vi "Actor Core.vi"(8 "error in":errorcluster, 11 "SLZ-KA1 in":refnum<class "SLZ-KA1.lvclass">) -> (0 "error out":errorcluster, 3 "Actor out":refnum<class "Actor.lvclass">)   [LabVIEW 2015, in "SLZ-KA1 Actor.lvlib" / "SLZ-KA1.lvclass"]
doc: "(<B>Filename</B>: Actor Framework.lvlib:Actor.lvclass:Actor Core.vi)\n\nReceives messages to the actor, reacts to them, and initiates any error handling that may shut the actor down.\n\nDescendant classes may override this VI to append parallel tasks for the actor to complete while it handles messages. Overrides use the Call Parent Method node."
uses:
  SLZ-KA1.lvclass
  <vilib>/ActorFramework/Actor/Actor.lvclass
  Controls/PV State Selector.ctl
  SLZ-KA1.lvclass/SLZ-KA1.ctl
  Controls/SLZ-KA1 Virtual Data Cluster.ctl
  Controls/SLZ-KA1 Real Data Cluster.ctl
  <vilib>/Modbus/master/Create Master Instance (TCP).vi
  <vilib>/Modbus/slave/Create Slave Instance (TCP).vi
  <vilib>/Modbus/slave/Modbus Slave.lvclass
  <vilib>/Modbus/master/Modbus Master.lvclass
  Utilities/Modbus Data Conversion.llb/Modbus Data Conversion.lvlib
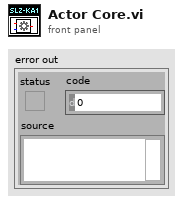
[diagram p1: front panel]
types:
  T1 = typedef "SLZ-KA1 Actor.lvlib/SLZ-KA1.lvclass/PV State Selector.ctl" = enum16{"Init", "Read", "Error Check", "Close"}
  T2 = typedef "SLZ-KA1 Actor.lvlib/SLZ-KA1.lvclass/SLZ-KA1 Real Data Cluster.ctl" = cluster{"Drive On/Off":enum16{"Off", "On"}, "Room Temperature":dbl, "Fault Code":u16}
  T3 = typedef "SLZ-KA1 Actor.lvlib/SLZ-KA1.lvclass/SLZ-KA1 Virtual Data Cluster.ctl" = cluster{"Drive Mode":u16, "Temperature Setpoint":dbl, "Drive On/Off":enum16{"Off", "On"}}
  T4 = cluster{"Drive Mode":bool, "Temperature Setpoint":bool, "Drive On/Off":bool}
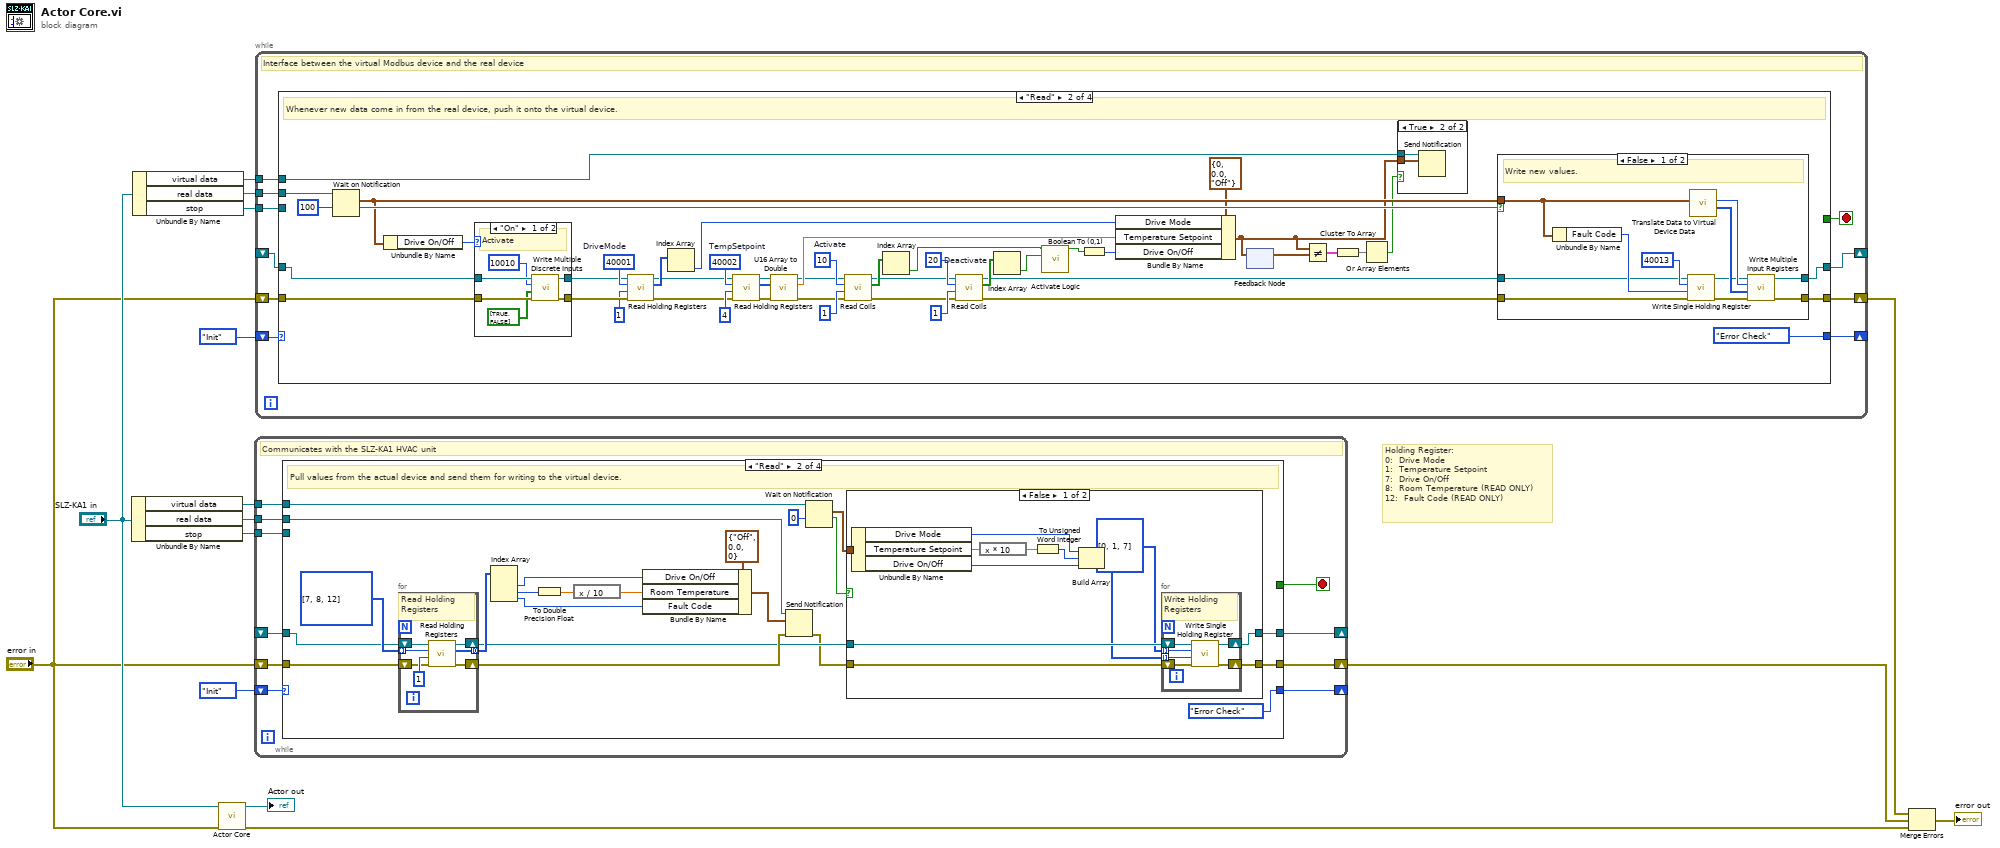
[diagram p0: block diagram]
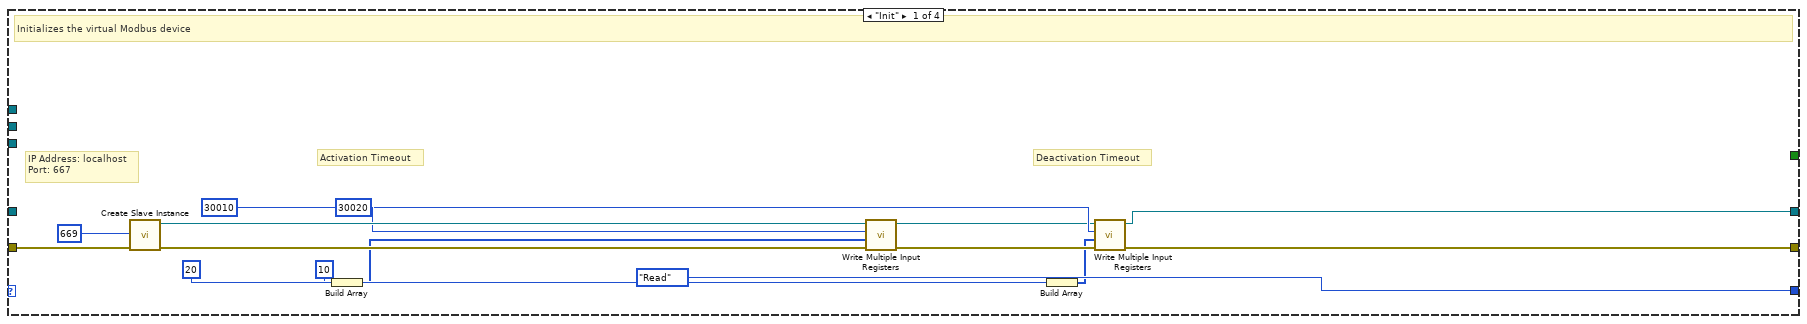
[diagram p2: hidden frame]
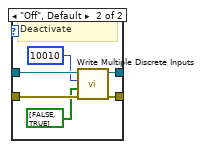
[diagram p5: hidden frame]
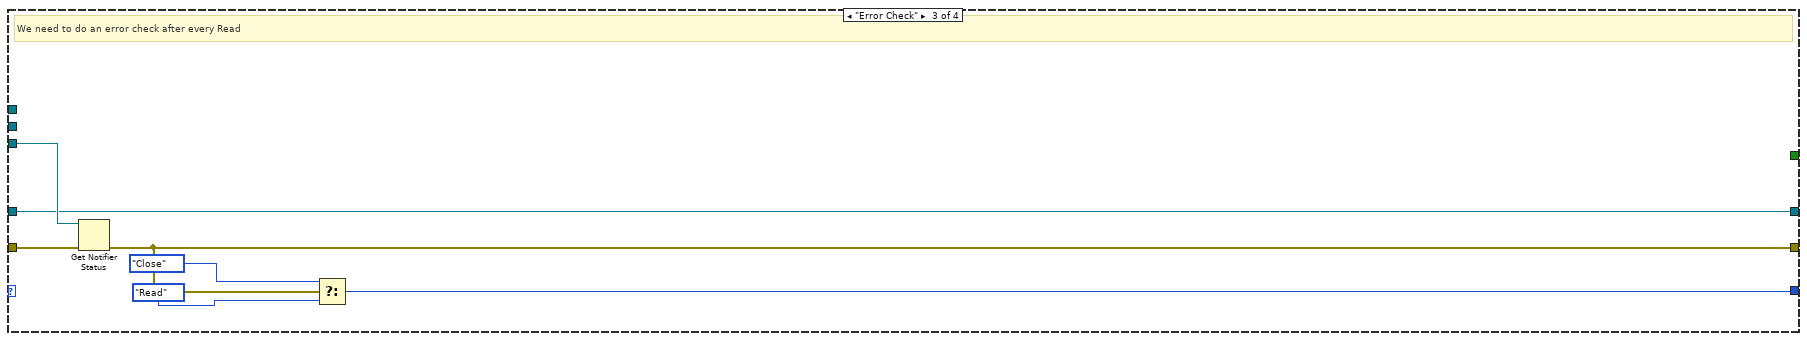
[diagram p6: hidden frame]
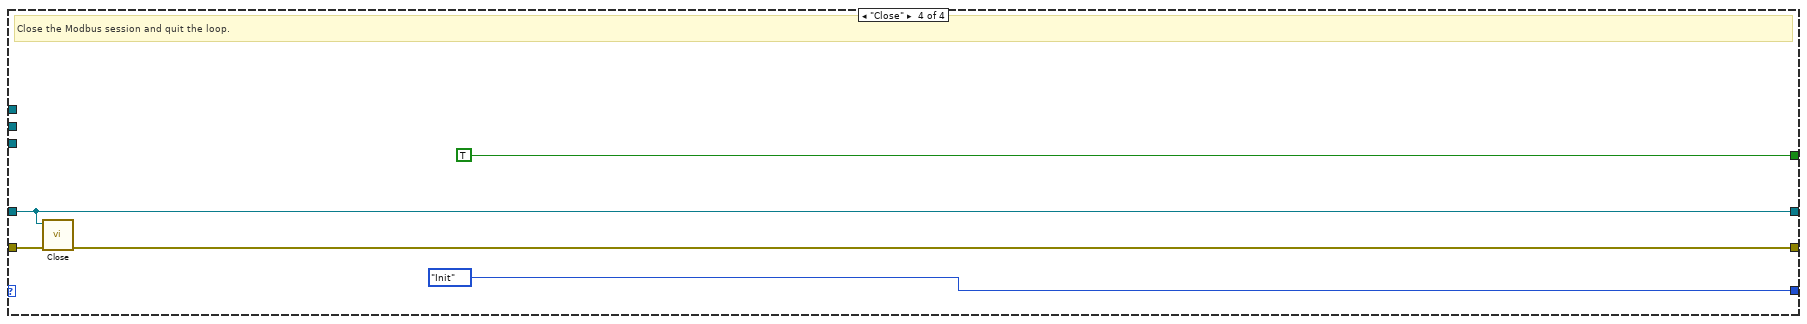
[diagram p7: hidden frame]
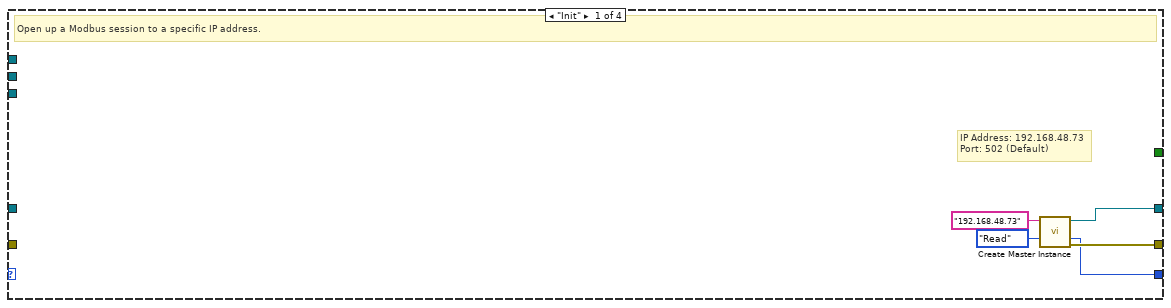
[diagram p8: hidden frame]
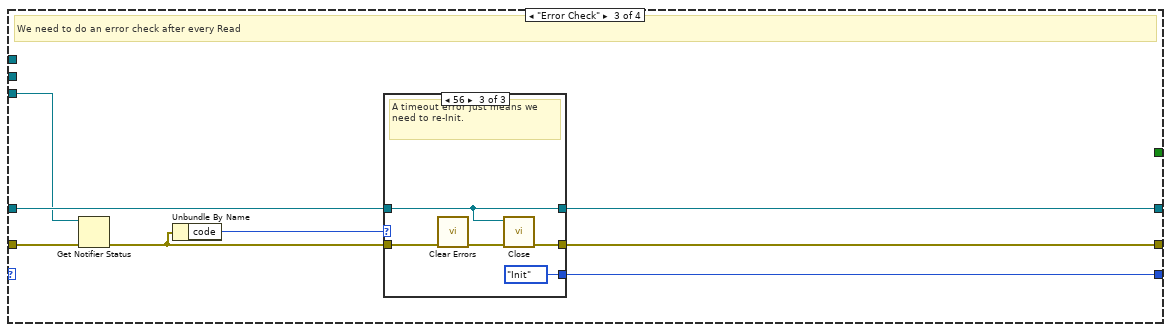
[diagram p10: hidden frame]
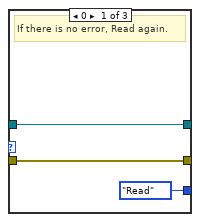
[diagram p11: hidden frame]
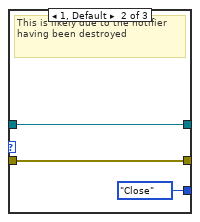
[diagram p12: hidden frame]
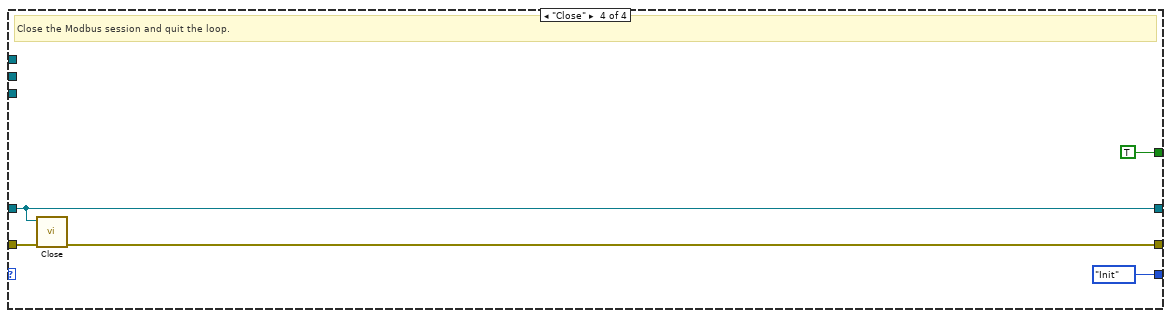
[diagram p13: hidden frame]
diagram:
  # "Holding Register:\n0:  Drive Mode\n1:  Temperature Setpoint\n7:  Drive On/Off\n8:  Room Temperature (READ ONLY)\n12:  Fault Code (READ ONLY)"
  n1 = Unbundle By Name("SLZ-KA1 in") -> ("virtual data"=w1:refnum<notifier>, "real data"=w12:refnum<notifier>, "stop"=w11:refnum<notifier>)
  n2 = Unbundle By Name("SLZ-KA1 in") -> ("virtual data"=w2:refnum<notifier>, "real data"=w5:refnum<notifier>, "stop"=w4:refnum<notifier>)
  n3 = call-parent "Actor Core.vi"("error in"="error in", "Actor in"="SLZ-KA1 in") -> ("error out"=w15:errorcluster, "Actor out"=→"Actor out":refnum<class "Actor.lvclass">)  [unwired: 8 in]
  n4 = while {
    shift-right: [w23] -> _
    shift-left: PV_State_Selector."Init" -> [w25]
    shift-right: [w24] -> _
    shift-left: _ -> [w22]
    shift-right: [w20] -> w9
    shift-left: "error in" -> [w21]
    tunnel: w12 -> [w19]
    tunnel: w11 -> [w17]
    tunnel: w1 -> [w16]
    stop <- w18 stop-if-true
    # "Communicates with the SLZ-KA1 HVAC unit"
    n5 = case shown="\"Read\"" w25 {
      tunnel: [w28 w34 w82 w99] -> w24
      tunnel: [w27 w32 w85 w101] -> w20
      tunnel: [PV_State_Selector."Read" PV_State_Selector."Error Check" w83 PV_State_Selector."Init"] -> w23
      tunnel: w22 -> [_ w47 w84 w99]
      tunnel: w21 -> [_ w48 w81 w102]
      tunnel: [_ _ _ TRUE ("stop")] -> w18
      tunnel: w19 -> [_ w50 _ _]
      tunnel: w17 -> [_ _ w79 _]
      tunnel: w16 -> [_ w37 _ _]
      frame "Init" {
        # "IP Address: 192.168.48.73\nPort: 502 (Default)"
        # "Open up a Modbus session to a specific IP address."
        n6 = call-poly <vilib>:"Create Master Instance.vi"("address"="192.168.48.73") -> ("error out"=w27:errorcluster, "TCP master instance"=w28:refnum<class "Modbus Master.lvclass">)  [unwired: 9 in]
      }
      frame "Read" {
        # "Pull values from the actual device and send them for writing to the virtual device."
        n7 = for {
          tunnel: [w74] -> w45 mode=concatenating
          shift-right: [w77] -> w35
          shift-left: w47 -> [w75]
          tunnel: u16[] [7, 8, 12] ("starting address") -> [w73] mode=indexing
          shift-right: [w76] -> w46
          shift-left: w48 -> [w72]
          # "Read Holding Registers"
          n8 = call-dynamic "Read Holding Registers.vi"("error in (no error)"=w72, "number of holding registers"=u16 1, "starting address"=w73, "Modbus master in"=w75) -> ("error out"=w76:errorcluster, "register values"=w74:u16[], "Modbus master out"=w77:refnum<class "Modbus Master.lvclass">)  [unwired: 5 in]
        }
        n9 = Index Array(array=w45) -> (element #1=w43:u16, element #2=w41:u16, element #3=w40:u16)  [unwired: 3 in]
        n10 = To Double Precision Float(number=w41) -> (double precision float=w31:dbl)
        n11 = expression code="x / 10"(w31) -> (w42:dbl)
        n12 = Bundle By Name(cluster=T2 {"Drive On/Off"=enum."Off", "Room Temperature"=0.0, "Fault Code"=0}, "Drive On/Off"=w43, "Room Temperature"=w42, "Fault Code"=w40) -> (w39:T2)
        n13 = Send Notification(notification=w39, notifier=w50, error in (no error)=w46) -> (error out=w33:errorcluster)  [unwired: 1 out]
        n14 = Wait on Notification(notifier=w37, timeout in ms (-1)=0) -> (notification=w36:T3, timed out?=w30:bool)  [unwired: 2 in, 2 out]
        n15 = case shown="False" w30 {
          tunnel: w36 -> [w63 _]
          tunnel: w35 -> [w62 w71]
          tunnel: [w61 w71] -> w34
          tunnel: w33 -> [w60 w70]
          tunnel: [w59 w70] -> w32
          frame False {
            n16 = Unbundle By Name(w63) -> ("Drive Mode"=w56:u16, "Temperature Setpoint"=w58:dbl, "Drive On/Off"=w54:enum16{"Off", "On"})
            n17 = expression code="x * 10"(w58) -> (w57:dbl)
            n18 = To Unsigned Word Integer(number=w57) -> (unsigned 16bit integer=w55:u16)
            n19 = Build Array(w56, w55, w54) -> (w53:u16[])
            n20 = for {
              shift-right: [w69] -> w61
              shift-left: w62 -> [w67]
              shift-right: [w68] -> w59
              shift-left: w60 -> [w66]
              tunnel: w53 -> [w65] mode=indexing
              tunnel: u16[] [0, 1, 7] ("starting address") -> [w64] mode=indexing
              # "Write Holding Registers"
              n21 = call-dynamic "Write Single Holding Register.vi"("error in (no error)"=w66, "holding register value"=w65, "address"=w64, "Modbus master in"=w67) -> ("error out"=w68:errorcluster, "Modbus master out"=w69:refnum<class "Modbus Master.lvclass">)  [unwired: 6 in]
            }
          }
          frame True {
          }
        }
      }
      frame "Error Check" {
        # "We need to do an error check after every Read"
        n22 = Get Notifier Status(notifier=w79, error in (no error)=w81) -> (error out=w80:errorcluster)  [unwired: 4 out]
        n23 = Unbundle By Name(w80) -> ("code"=w86:i32)
        n24 = case shown="56" w86 {
          tunnel: w80 -> [w89 w90 w97]
          tunnel: [w89 w90 w95] -> w85
          tunnel: w84 -> [w88 w91 w93]
          tunnel: [PV_State_Selector."Read" PV_State_Selector."Close" PV_State_Selector."Init"] -> w83
          tunnel: [w88 w91 w93] -> w82
          frame 0 {
            # "If there is no error, Read again."
          }
          frame 1, Default {
            # "This is likely due to the notifier having been destroyed"
          }
          frame 56 {
            # "A timeout error just means we need to re-Init."
            n25 = call <vilib>:"Clear Errors.vi"("error in (no error)"=w97) -> ("error out"=w96:errorcluster)  [unwired: 5 in, 1 out]
            n26 = call-dynamic "Close.vi"("error in (no error)"=w96, "Modbus master in"=w93) -> ("error out"=w95:errorcluster)  [unwired: 9 in]
          }
        }
      }
      frame "Close" {
        # "Close the Modbus session and quit the loop."
        n27 = call-dynamic "Close.vi"("error in (no error)"=w102, "Modbus master in"=w99) -> ("error out"=w101:errorcluster)  [unwired: 9 in]
      }
    }
  }
  n28 = while {
    shift-right: [w112] -> _
    shift-left: _ -> [w108]
    shift-right: [w111] -> w3
    shift-left: "error in" -> [w107]
    tunnel: w5 -> [w106]
    tunnel: w4 -> [w105]
    shift-right: [w104] -> _
    shift-left: PV_State_Selector."Init" -> [w110]
    tunnel: w2 -> [w103]
    stop <- w109 stop-if-true
    # "Interface between the virtual Modbus device and the real device"
    n29 = case shown="\"Read\"" w110 {
      tunnel: [w115 w166 w201 w207] -> w112
      tunnel: [w114 w167 w202 w208] -> w111
      tunnel: [PV_State_Selector."Read" PV_State_Selector."Error Check" w203 PV_State_Selector."Init"] -> w104
      tunnel: [_ _ _ TRUE ("stop")] -> w109
      tunnel: w108 -> [_ w158 w201 w207]
      tunnel: w107 -> [w113 w157 w200 w209]
      tunnel: w106 -> [_ w171 _ _]
      tunnel: w105 -> [_ _ w206 _]
      tunnel: w103 -> [_ w156 _ _]
      frame "Init" {
        # "Deactivation Timeout"
        # "Activation Timeout"
        # "IP Address: localhost\nPort: 667"
        # "Initializes the virtual Modbus device"
        n30 = call-poly <vilib>:"Create Slave Instance.vi"("error in (no error)"=w113, "port (502)"=u16 669) -> ("error out"=w124:errorcluster, "TCP slave instance"=w125:refnum<class "Modbus Slave.lvclass">)  [unwired: 8 in]
        n31 = Build Array(u16 20 ("Register")) -> (w117:u16[])
        n32 = call-dynamic "Write Multiple Input Registers.vi"("error in (no error)"=w124, "input register values"=w117, "starting address"=u16 30010, "Modbus slave in"=w125) -> ("error out"=w120:errorcluster, "Modbus slave out"=w121:refnum<class "Modbus Slave.lvclass">)  [unwired: 6 in]
        n33 = Build Array(u16 10 ("Register")) -> (w116:u16[])
        n34 = call-dynamic "Write Multiple Input Registers.vi"("error in (no error)"=w120, "input register values"=w116, "starting address"=u16 30020, "Modbus slave in"=w121) -> ("error out"=w114:errorcluster, "Modbus slave out"=w115:refnum<class "Modbus Slave.lvclass">)  [unwired: 6 in]
      }
      frame "Read" {
        w147 = u16 40002  # TempSetpoint
        w154 = u16 40001  # DriveMode
        w163 = u16 20  # Deactivate
        w170 = u16 10  # Activate
        # "Whenever new data come in from the real device, push it onto the virtual device."
        n35 = Wait on Notification(notifier=w171, timeout in ms (-1)=100) -> (notification=w159:T2, timed out?=w161:bool)  [unwired: 2 in, 2 out]
        n36 = Unbundle By Name(w159) -> ("Drive On/Off"=w160:enum16{"Off", "On"})
        n37 = case shown="\"On\"" w160 {
          tunnel: w157 -> [w192 w198]
          tunnel: w158 -> [w193 w199]
          tunnel: [w189 w195] -> w153
          tunnel: [w188 w194] -> w152
          frame "On" {
            # "Activate"
            n38 = call-dynamic "Write Multiple Discrete Inputs.vi"("error in (no error)"=w192, "discrete input values"=bool[] [TRUE, FALSE], "starting address"=u16 10010, "Modbus slave in"=w193) -> ("error out"=w188:errorcluster, "Modbus slave out"=w189:refnum<class "Modbus Slave.lvclass">)  [unwired: 6 in]
          }
          frame "Off", Default {
            # "Deactivate"
            n39 = call-dynamic "Write Multiple Discrete Inputs.vi"("error in (no error)"=w198, "discrete input values"=bool[] [FALSE, TRUE], "starting address"=u16 10010, "Modbus slave in"=w199) -> ("error out"=w194:errorcluster, "Modbus slave out"=w195:refnum<class "Modbus Slave.lvclass">)  [unwired: 6 in]
          }
        }
        n40 = call-dynamic "Read Holding Registers.vi"("error in (no error)"=w152, "number of holding registers"=u16 1, "starting address"=w154, "Modbus slave in"=w153) -> ("error out"=w145:errorcluster, "register values"=w150:u16[], "Modbus slave out"=w146:refnum<class "Modbus Slave.lvclass">)  [unwired: 5 in]
        n41 = Index Array(array=w150) -> (element=w149:u16)  [unwired: 1 in]
        n42 = call-dynamic "Read Holding Registers.vi"("error in (no error)"=w145, "number of holding registers"=u16 4, "starting address"=w147, "Modbus slave in"=w146) -> ("error out"=w141:errorcluster, "register values"=w144:u16[], "Modbus slave out"=w142:refnum<class "Modbus Slave.lvclass">)  [unwired: 5 in]
        n43 = call "U16 Array to Double.vi"("U16 Array"=w144) -> ("Double"=w143:dbl)  [unwired: 10 in]
        n44 = call-dynamic "Read Coils.vi"("error in (no error)"=w141, "number of coils"=u16 1, "starting address"=w170, "Modbus slave in"=w142) -> ("error out"=w139:errorcluster, "coil values"=w168:bool[], "Modbus slave out"=w140:refnum<class "Modbus Slave.lvclass">)  [unwired: 5 in]
        n45 = Index Array(array=w168) -> (element=w134:bool)  [unwired: 1 in]
        n46 = call-dynamic "Read Coils.vi"("error in (no error)"=w139, "number of coils"=u16 1, "starting address"=w163, "Modbus slave in"=w140) -> ("error out"=w136:errorcluster, "coil values"=w165:bool[], "Modbus slave out"=w137:refnum<class "Modbus Slave.lvclass">)  [unwired: 5 in]
        n47 = Index Array(array=w165) -> (element=w133:bool)  [unwired: 1 in]
        n48 = call "Activate Logic.vi"("Deactivate"=w133, "Activate"=w134) -> ("Output"=w135:bool)  [unwired: 9 in]
        n49 = Boolean To (0,1)(Boolean=w135) -> (0, 1=w138:i16)
        n50 = Bundle By Name(cluster=T3 {"Drive Mode"=0, "Temperature Setpoint"=0.0, "Drive On/Off"=enum."Off"} ("notification"), "Drive Mode"=w149, "Temperature Setpoint"=w143, "Drive On/Off"=w138) -> (w131:T3)
        n51 = feedback-in #1(w131) -> ()
        n52 = feedback #1() -> (w132:T3)  [unwired: 1 in]
        n53 = Not Equal?(x=w131, y=w132) -> (x != y?=w130:T4)
        n54 = Cluster To Array(cluster=w130) -> (array=w129:bool[])
        n55 = Or Array Elements(Boolean array=w129) -> (logical OR=w128:bool)
        n56 = case shown="True" w128 {
          tunnel: w156 -> [_ w174]
          tunnel: w131 -> [_ w173]
          frame False {
          }
          frame True {
            n57 = Send Notification(notification=w173, notifier=w174) -> ()  [unwired: 1 in, 2 out]
          }
        }
        n58 = case shown="False" w161 {
          tunnel: w159 -> [w181 _]
          tunnel: w136 -> [w178 w186]
          tunnel: [w183 w186] -> w167
          tunnel: [w182 w187] -> w166
          tunnel: w137 -> [w176 w187]
          frame False {
            # "Write new values."
            n59 = Unbundle By Name(w181) -> ("Fault Code"=w179:u16)
            n60 = call-dynamic "Write Single Holding Register.vi"("error in (no error)"=w178, "holding register value"=w179, "address"=u16 40013 ("starting address"), "Modbus slave in"=w176) -> ("error out"=w177:errorcluster, "Modbus slave out"=w175:refnum<class "Modbus Slave.lvclass">)  [unwired: 6 in]
            n61 = call "Translate Data to Virtual Device Data.vi"("HVAC Data"=w181) -> ("Data Array"=w184:u16[], "Address"=w185:u16)  [unwired: 9 in]
            n62 = call-dynamic "Write Multiple Input Registers.vi"("error in (no error)"=w177, "input register values"=w184, "starting address"=w185, "Modbus slave in"=w175) -> ("error out"=w183:errorcluster, "Modbus slave out"=w182:refnum<class "Modbus Slave.lvclass">)  [unwired: 6 in]
          }
          frame True {
            # "Don't write new values on a timeout."
          }
        }
      }
      frame "Error Check" {
        # "We need to do an error check after every Read"
        n63 = Get Notifier Status(notifier=w206, error in (no error)=w200) -> (error out=w202:errorcluster)  [unwired: 4 out]
        n64 = Select(t=PV_State_Selector."Close", s=w202, f=PV_State_Selector."Read") -> (s? t:f=w203:T1)
      }
      frame "Close" {
        # "Close the Modbus session and quit the loop."
        n65 = call-dynamic "Close.vi"("error in (no error)"=w209, "Modbus slave in"=w207) -> ("error out"=w208:errorcluster)  [unwired: 9 in]
      }
    }
  }
  n66 = Merge Errors(w3, w9, w15) -> (→"error out":errorcluster)
